vi "ZeroMQ_SUBGS.vi"() -> ()   [LabVIEW 2018]
uses:
  <vilib>/addons/zeromq/socket_type.ctl
  <vilib>/addons/zeromq/socket_options.ctl
  <vilib>/addons/zeromq/zeromq.lvlib
  <vilib>/addons/zeromq/zmq_socket.lvclass
  <vilib>/addons/zeromq/zmq_context.lvclass
panel:
  out "error out 2":errorcluster
  out "message":string
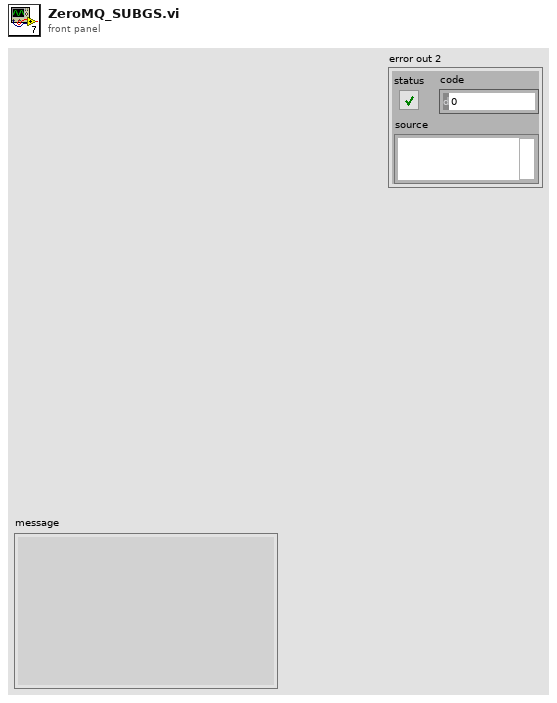
[diagram p1: front panel]
types:
  T1 = cluster{"ID":u32, "Address":string, "Service Name 1":string, "Service Name 2":string, "queue TX":refnum<queue>, "queue RX":refnum<queue>, "Port 1":u32, "Port 2":u32}
  T2 = typedef "zeromq.lvlib/socket_options.ctl" = enum8{"NONE", "ZMQ_HWM", "<2>", "ZMQ_SWAP", "ZMQ_AFFINITY", "ZMQ_ROUTING_ID", "ZMQ_SUBSCRIBE", "ZMQ_UNSUBSCRIBE", "ZMQ_RATE", "ZMQ_RECOVERY_IVL", "ZMQ_MCAST_LOOP", "ZMQ_SNDBUF", "ZMQ_RCVBUF", "ZMQ_RCVMORE", "ZMQ_FD", "ZMQ_EVENTS", "ZMQ_TYPE", "ZMQ_LINGER", "ZMQ_RECONNECT_IVL", "ZMQ_BACKLOG", "ZMQ_RECOVERY_IVL_MSEC", "ZMQ_RECONNECT_IVL_MAX", "ZMQ_MAXMSGSIZE", "ZMQ_SNDHWM", "ZMQ_RCVHWM", "ZMQ_MULTICAST_HOPS", "<26>", "ZMQ_RCVTIMEO", "ZMQ_SNDTIMEO", "<29>", "<30>", "ZMQ_IPV4ONLY", "ZMQ_LAST_ENDPOINT", "ZMQ_ROUTER_MANDATORY", "ZMQ_TCP_KEEPALIVE", "ZMQ_TCP_KEEPALIVE_CNT", "ZMQ_TCP_KEEPALIVE_IDLE", "ZMQ_TCP_KEEPALIVE_INTVL", "ZMQ_TCP_ACCEPT_FILTER", "ZMQ_IMMEDIATE", "ZMQ_XPUB_VERBOSE", "ZMQ_ROUTER_RAW", "ZMQ_IPV6", "ZMQ_MECHANISM", "ZMQ_PLAIN_SERVER", "ZMQ_PLAIN_USERNAME", "ZMQ_PLAIN_PASSWORD", "ZMQ_CURVE_SERVER", "ZMQ_CURVE_PUBLICKEY", "ZMQ_CURVE_SECRETKEY", "ZMQ_CURVE_SERVERKEY", "ZMQ_PROBE_ROUTER", "ZMQ_REQ_CORRELATE", "ZMQ_REQ_RELAXED", "ZMQ_CONFLATE", "ZMQ_ZAP_DOMAIN", "ZMQ_ROUTER_HANDOVER", "ZMQ_TOS", "ZMQ_IPC_FILTER_PID", "ZMQ_IPC_FILTER_UID", "ZMQ_IPC_FILTER_GID", "ZMQ_CONNECT_ROUTING_ID", "ZMQ_GSSAPI_SERVER", "ZMQ_GSSAPI_PRINCIPAL", "ZMQ_GSSAPI_SERVICE_PRINCIPAL", "ZMQ_GSSAPI_PLAINTEXT", "ZMQ_HANDSHAKE_IVL", "<67>", "ZMQ_SOCKS_PROXY", "ZMQ_XPUB_NODROP", "ZMQ_BLOCKY", "ZMQ_XPUB_MANUAL", "ZMQ_XPUB_WELCOME_MSG", "ZMQ_STREAM_NOTIFY", "ZMQ_INVERT_MATCHING", "ZMQ_HEARTBEAT_IVL", "ZMQ_HEARTBEAT_TTL", "ZMQ_HEARTBEAT_TIMEOUT", "ZMQ_XPUB_VERBOSER", "ZMQ_CONNECT_TIMEOUT", "ZMQ_TCP_MAXRT", "ZMQ_THREAD_SAFE", "<82>", "<83>", "ZMQ_MULTICAST_MAXTPDU", "ZMQ_VMCI_BUFFER_SIZE", "ZMQ_VMCI_BUFFER_MIN_SIZE", "ZMQ_VMCI_BUFFER_MAX_SIZE", "ZMQ_VMCI_CONNECT_TIMEOUT", "ZMQ_USE_FD", "ZMQ_GSSAPI_PRINCIPAL_NAMETYPE", "ZMQ_GSSAPI_SERVICE_PRINCIPAL_NAMETYPE", "ZMQ_BINDTODEVICE", "ZMQ_ZAP_ENFORCE_DOMAIN", "ZMQ_LOOPBACK_FASTPATH", "ZMQ_METADATA", "ZMQ_MULTICAST_LOOP", "ZMQ_ROUTER_NOTIFY"}
  T3 = typedef "zeromq.lvlib/socket_type.ctl" = enum8{"ZMQ_PAIR", "ZMQ_PUB", "ZMQ_SUB", "ZMQ_REQ", "ZMQ_REP", "ZMQ_DEALER", "ZMQ_ROUTER", "ZMQ_PULL", "ZMQ_PUSH", "ZMQ_XPUB", "ZMQ_XSUB", "ZMQ_STREAM", "ZMQ_SERVER", "ZMQ_CLIENT", "ZMQ_RADIO", "ZMQ_DISH", "ZMQ_GATHER", "ZMQ_SCATTER", "ZMQ_DGRAM"}
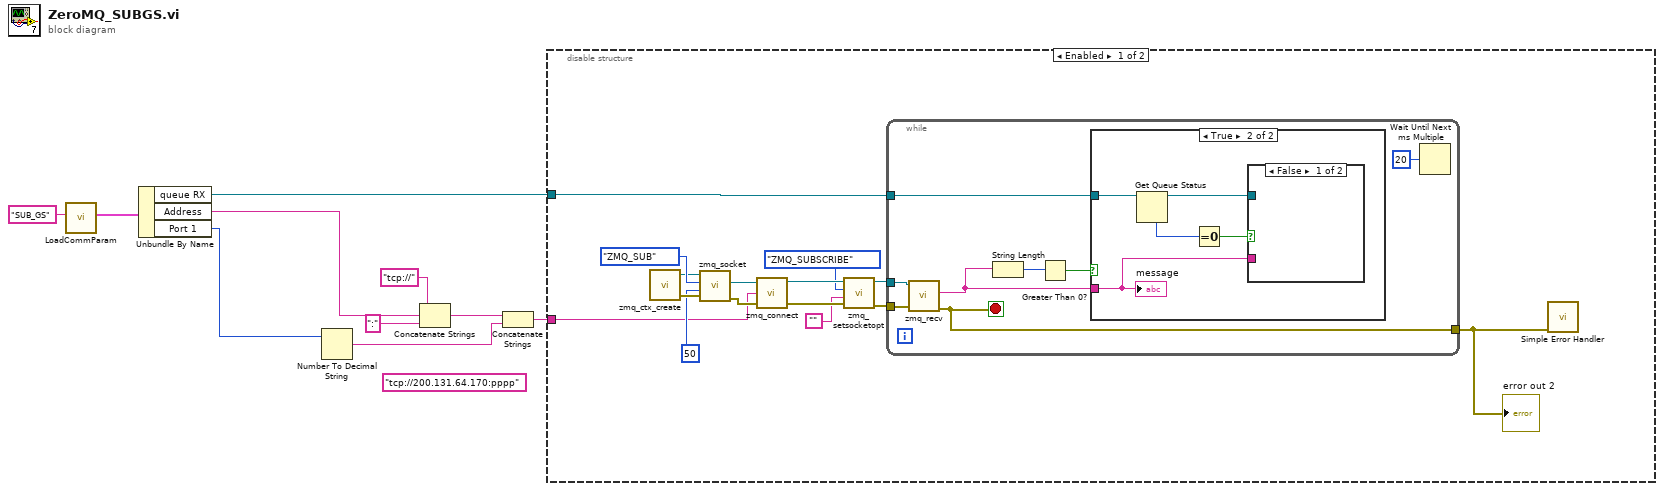
[diagram p0: block diagram]
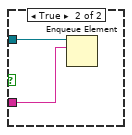
[diagram p3: hidden frame]
diagram:
  (unwired) "tcp://200.131.64.170:pppp" ("endpoint")
  n1 = call "LoadCommParam.vi"("section name"="SUB_GS") -> ("output cluster"=w1:T1)  [unwired: 10 in]
  n2 = Unbundle By Name(w1) -> ("queue RX"=w2:refnum<queue>, "Address"=w9:string, "Port 1"=w8:u32)
  n3 = Number To Decimal String(number=w8) -> (decimal integer string=w7:string)  [unwired: 1 in]
  n4 = Concatenate Strings("tcp://" ("string"), w9, ":" ("string")) -> (w6:string)
  n5 = Concatenate Strings(w6, w7) -> (w3:string)
  n6 = disable-structure shown="Enabled" {
    disable-tunnel: w2 -> [w12 _]
    disable-tunnel: w3 -> [w11 _]
    frame Enabled {
      n7 = call <vilib>:"zmq_ctx_create.vi"() -> ("error out"=w24:errorcluster, "context out"=w14:refnum<class "zmq_context.lvclass">)  [unwired: 4 in]
      n8 = call <vilib>:"zmq_socket.vi"("error in"=w24, "linger (ms)"=50, "socket type"=socket_type."ZMQ_SUB", "context in"=w14) -> ("error out"=w23:errorcluster, "socket out"=w15:refnum<class "zmq_socket.lvclass">)  [unwired: 1 in, 1 out]
      n9 = call <vilib>:"zmq_connect.vi"("error in"=w23, "endpoint"=w11, "socket in"=w15) -> ("error out"=w21:errorcluster, "socket out"=w22:refnum<class "zmq_socket.lvclass">)  [unwired: 1 in]
      n10 = call <vilib>:"zmq_setsocketopt.vi"("error in"=w21, "value"="", "option"=socket_options."ZMQ_SUBSCRIBE", "socket in"=w22) -> ("error out"=w20:errorcluster, "socket out"=w19:refnum<class "zmq_socket.lvclass">)  [unwired: 2 in]
      n11 = while {
        tunnel: w19 -> [w31]
        tunnel: w20 -> [w33]
        tunnel: [w32] -> w16
        tunnel: w12 -> [w28]
        stop <- w32 stop-if-true
        n12 = call <vilib>:"zmq_recv.vi"("error in"=w33, "socket in"=w31) -> ("error out"=w32:errorcluster, "data"=w27:string)  [unwired: 3 in, 3 out]
        n13 = String Length(string=w27) -> (length=w30:i32)
        n14 = Greater Than 0?(x=w30) -> (x > 0?=w29:bool)
        n15 = case shown="True" w29 {
          tunnel: w28 -> [_ w37]
          tunnel: w27 -> [_ w34]
          frame False {
          }
          frame True {
            n16 = Get Queue Status(queue=w37) -> (queue out=w35:refnum<queue>, # elements in queue=w38:i32)  [unwired: 2 in, 6 out]
            n17 = Equal To 0?(x=w38) -> (x = 0?=w36:bool)
            n18 = case shown="False" w36 {
              tunnel: w35 -> [_ w40]
              tunnel: w34 -> [_ w39]
              frame False {
              }
              frame True {
                n19 = Enqueue Element(queue=w40, element=w39) -> ()  [unwired: 2 in, 3 out]
              }
            }
            "message" <- w34
          }
        }
        n20 = Wait Until Next ms Multiple(millisecond multiple=u32 20) -> ()  [unwired: 1 out]
      }
      "error out 2" <- w16
      n21 = call <vilib>:"Simple Error Handler.vi"("error in (no error)"=w16) -> ()  [unwired: 4 in, 5 out]
    }
    frame Disabled {
    }
  }
